vi "Laser Controller.vi"(8 "error in (no error)":errorcluster, 10 "Notifiers":T1, 11 "All Message Queue Cluster":T2) -> (0 "error out":errorcluster)   [LabVIEW 2017]
uses:
  Lib QMH/AllMessageQueue Cluster.ctl
  Lib QMH/Message Cluster.ctl
  Lib Notifier/Notifier.ctl
  PulsePickerValues.ctl
  Lib QMH/MessageQueues.lvlib
  Lib Log/Logging.lvlib
  Lib Notifier/Notifier.lvlib
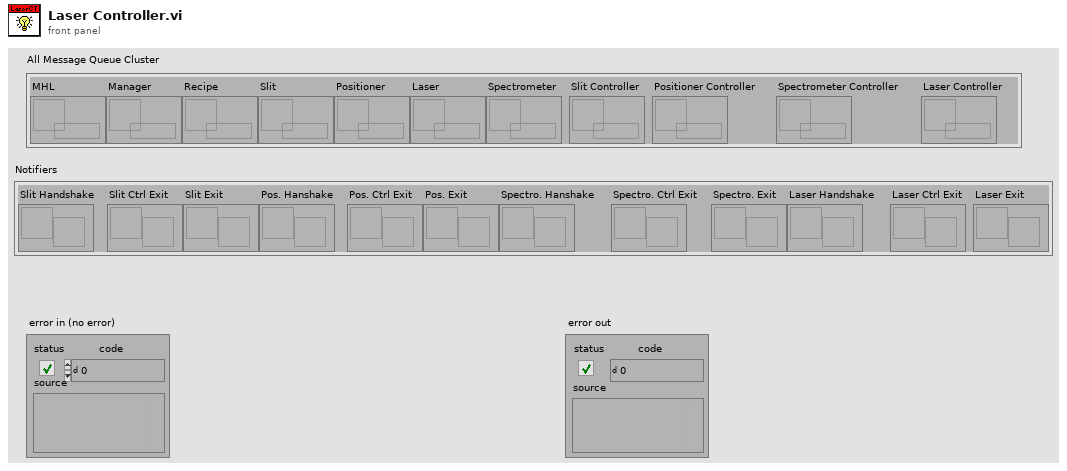
[diagram p1: front panel]
types:
  T1 = typedef "Notifier.lvlib/Notifier.ctl" = cluster{"Slit Handshake":refnum<notifier>, "Slit Ctrl Exit":refnum<notifier>, "Slit Exit":refnum<notifier>, "Pos. Hanshake":refnum<notifier>, "Pos. Ctrl Exit":refnum<notifier>, "Pos. Exit":refnum<notifier>, "Spectro. Hanshake":refnum<notifier>, "Spectro. Ctrl Exit":refnum<notifier>, "Spectro. Exit":refnum<notifier>, "Laser Handshake":refnum<notifier>, "Laser Ctrl Exit":refnum<notifier>, "Laser Exit":refnum<notifier>}
  T2 = typedef "MessageQueues.lvlib/AllMessageQueue Cluster.ctl" = cluster{"MHL":refnum<queue>, "Manager":refnum<queue>, "Recipe":refnum<queue>, "Slit":refnum<queue>, "Positioner":refnum<queue>, "Laser":refnum<queue>, "Spectrometer":refnum<queue>, "Slit Controller":refnum<queue>, "Positioner Controller":refnum<queue>, "Spectrometer Controller":refnum<queue>, "Laser Controller":refnum<queue>}
  T3 = enum16{"open", "replace", "create", "open or create", "replace or create", "replace or create with confirmation"}
  T4 = cluster{"état":bool, "code":i32, "source":string}
  T5 = typedef "PulsePickerValues.ctl" = u16
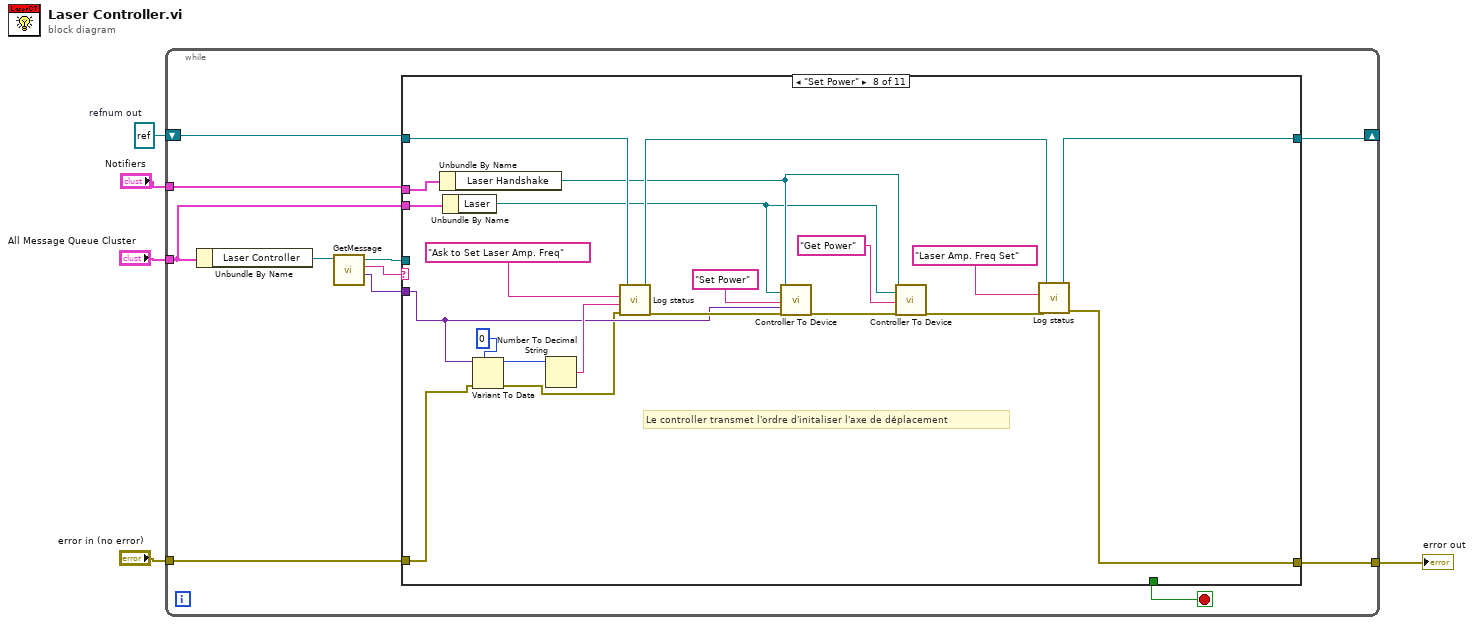
[diagram p0: block diagram]
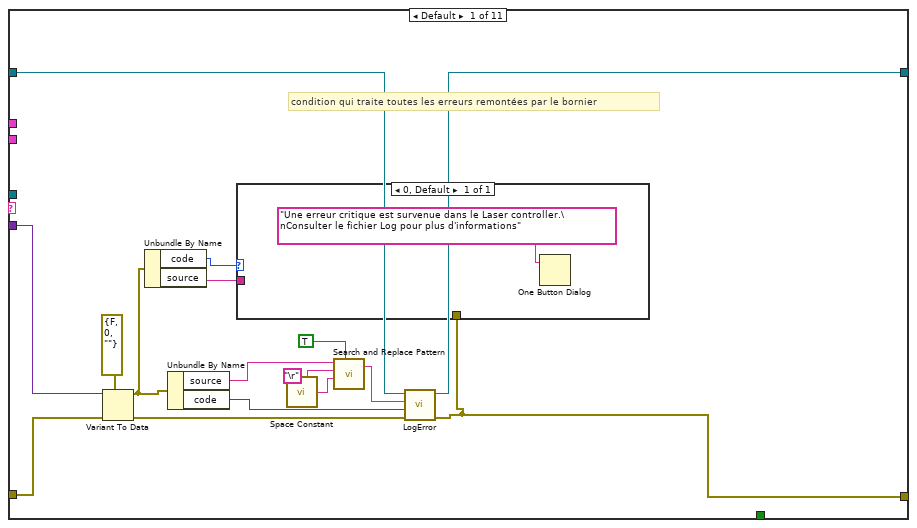
[diagram p2: hidden frame]
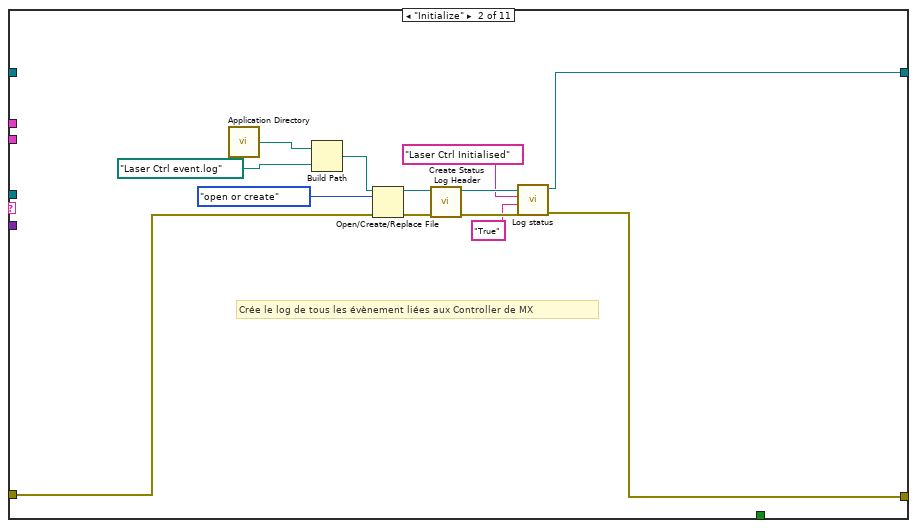
[diagram p3: hidden frame]
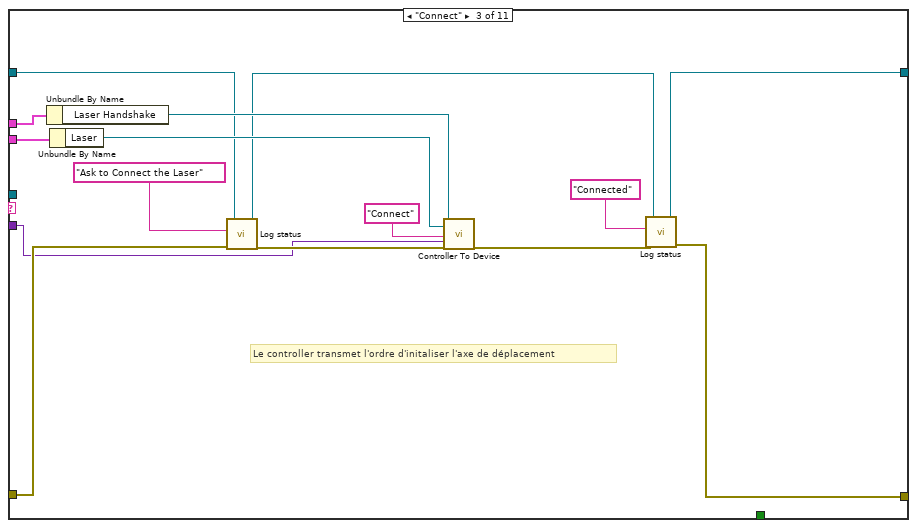
[diagram p4: hidden frame]
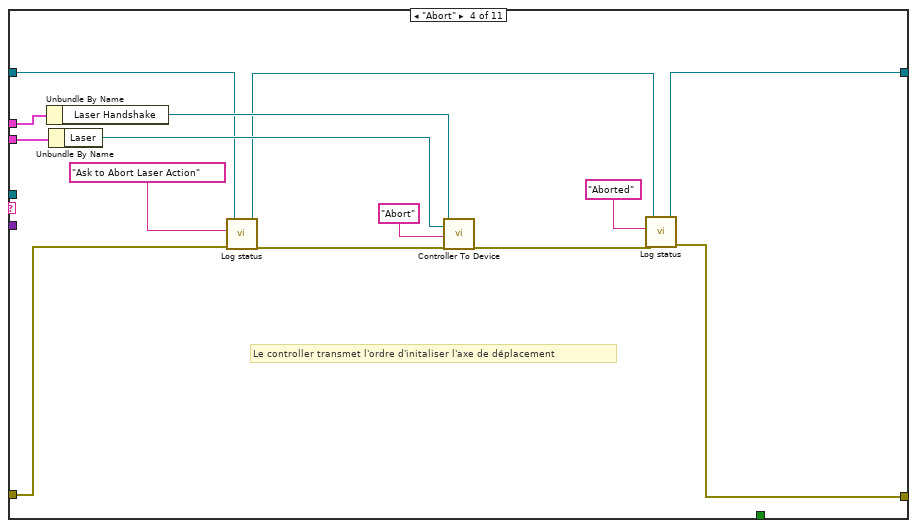
[diagram p5: hidden frame]
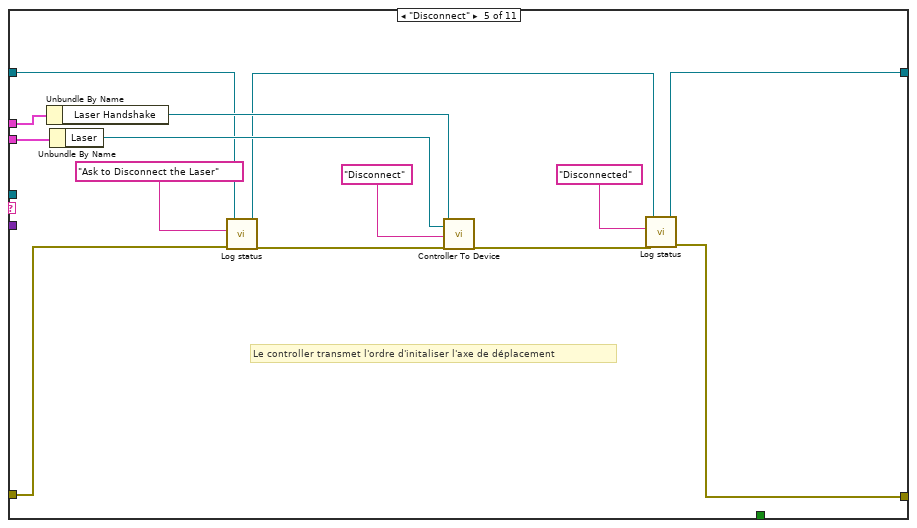
[diagram p6: hidden frame]
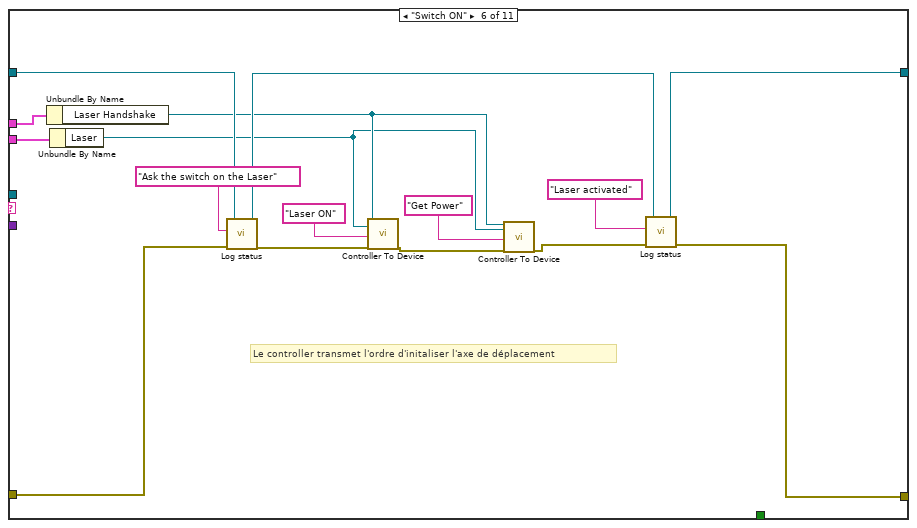
[diagram p7: hidden frame]
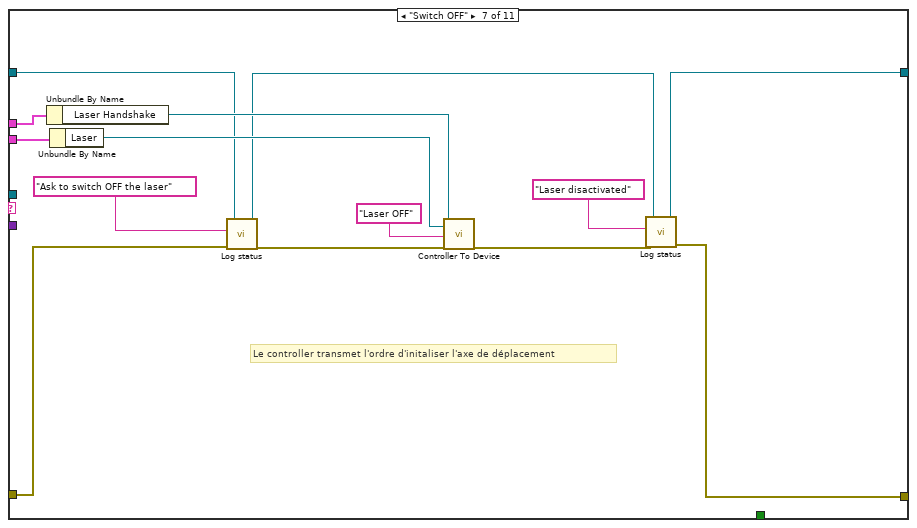
[diagram p8: hidden frame]
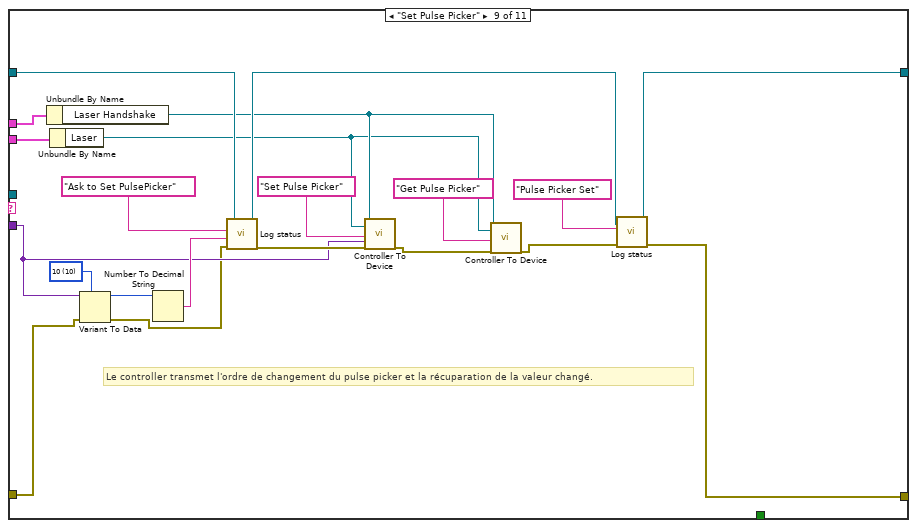
[diagram p9: hidden frame]
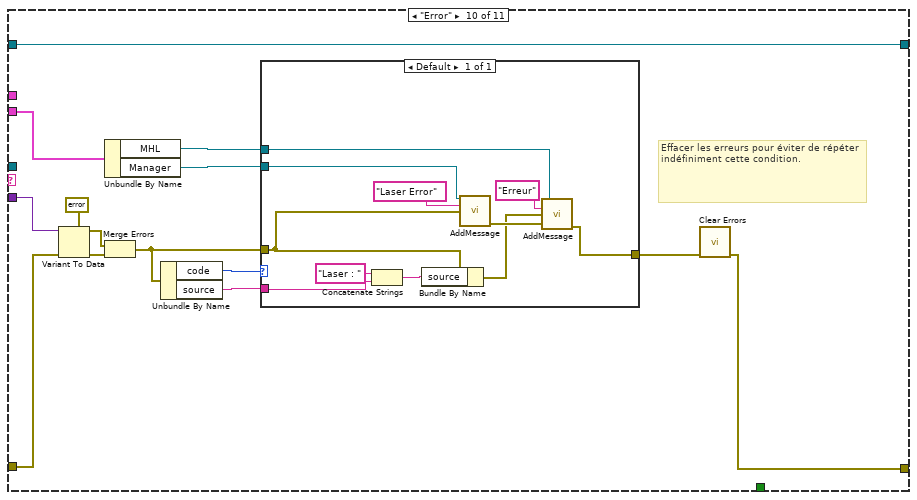
[diagram p10: hidden frame]
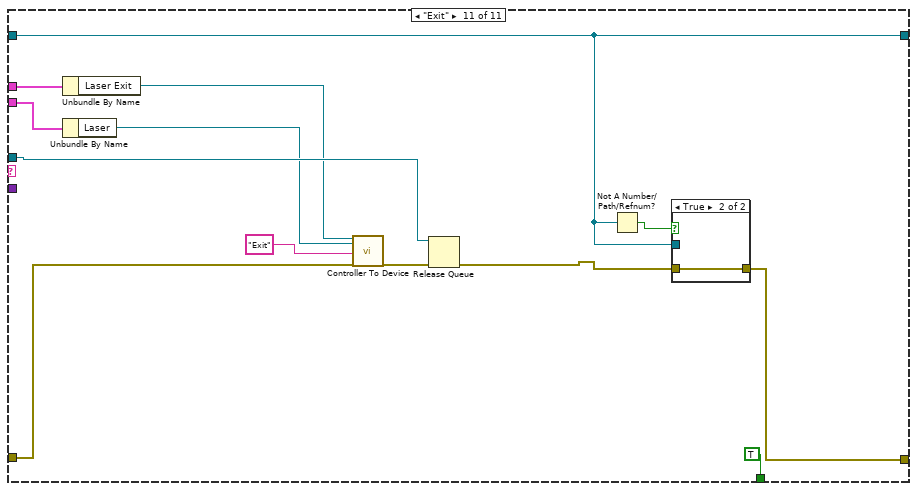
[diagram p11: hidden frame]
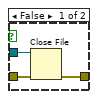
[diagram p12: hidden frame]
diagram:
  w2 = refnum<file> refnum  # refnum out
  n1 = while {
    tunnel: "All Message Queue Cluster" -> [w10]
    tunnel: "Notifiers" -> [w9]
    tunnel: "error in (no error)" -> [w8]
    tunnel: [w15] -> w1
    shift-right: [w12] -> _
    shift-left: w2 -> [w13]
    stop <- w14 stop-if-true
    n2 = Unbundle By Name(w10) -> ("Laser Controller"=w16:refnum<queue>)
    n3 = call "GetMessage.vi"("Message queue"=w16) -> ("Data"=w7:variant, "Message"=w6:string, "Dup Message Queue"=w11:refnum<queue>)  [unwired: 7 in, 1 out]
    n4 = case shown="\"Set Power\"" w6 {
      tunnel: w9 -> [_ _ w61 w75 w89 w105 w119 w140 w161 _ w196]
      tunnel: w10 -> [_ _ w60 w74 w88 w104 w118 w139 w160 w164 w195]
      tunnel: w8 -> [w21 w36 w49 w63 w77 w96 w107 w126 w149 w166 w191]
      tunnel: [_ _ _ _ _ _ _ _ _ _ TRUE] -> w14
      tunnel: w11 -> [_ _ _ _ _ _ _ _ _ _ w197]
      tunnel: w7 -> [w19 _ w47 _ _ _ _ w127 w150 w167 _]
      tunnel: [w17 w34 w52 w66 w80 w99 w110 w134 w155 w175 w193] -> w12
      tunnel: w13 -> [w18 _ w56 w70 w84 w102 w114 w137 w158 w175 w193]
      tunnel: [w20 w35 w54 w68 w82 w101 w112 w136 w157 w165 w194] -> w15
      frame Default {
        # "condition qui traite toutes les erreurs remontées par le bornier"
        n5 = Variant To Data(error in=w21, type=errorcluster {"status"=FALSE, "code"=0, "source"=""} ("error in (no error)"), Variant=w19) -> (data=w32:errorcluster, error out=w23:errorcluster)
        n6 = Unbundle By Name(w32) -> ("code"=w30:i32, "source"=w31:string)
        n7 = Unbundle By Name(w32) -> ("source"=w25:string, "code"=w24:i32)
        n8 = call <vilib>:"Space Constant.vi"() -> ("String"=w27:string)
        n9 = call <vilib>:"Search and Replace Pattern.vi"("string"=w25, "regular expression (\"\")"="\r", "replace string (\"\")"=w27, "replace all? (F)"=TRUE) -> ("result string"=w28:string)  [unwired: 1 in, 1 out]
        n10 = call "LogError.vi"("entrée d'erreur"=w23, "Code"=w24, "Source"=w28, "Error log refnum In"=w18) -> ("error out"=w20:errorcluster, "Error log refnum out"=w17:refnum<file>)  [unwired: 6 in]
        n11 = case shown="0, Default" w30 {
          tunnel: w31 -> [_]
          tunnel: w20 -> [_]
          frame 0, Default {
            n12 = One Button Dialog(message="Une erreur critique est survenue dans le Laser controller.\nConsulter le fichier Log pour plus d'informations" ("chaîne de format")) -> ()  [unwired: 1 in, 1 out]
          }
        }
      }
      frame "Initialize" {
        # "Crée le log de tous les évènement liées aux Controller de MX"
        n13 = call <vilib>:"Application Directory.vi"() -> ("Application Directory"=w43:path)
        n14 = Build Path(base path=w43, name or relative path=path "Laser Ctrl event.log") -> (appended path=w45:path)
        n15 = Open/Create/Replace File(file path (use dialog)=w45, error in=w36, operation (0:open)=T3."open or create" ("opération (0 : open)")) -> (refnum out=w41:refnum<file>, error out=w42:errorcluster)  [unwired: 3 in, 1 out]
        n16 = call "Create Status Log Header.vi"("entrée d'erreur"=w42, "Log File Refnum In"=w41) -> ("sortie d'erreur"=w40:errorcluster, "Log File Refnum out"=w39:refnum<file>)  [unwired: 8 in]
        n17 = call "Log status.vi"("entrée d'erreur"=w40, "Event Data String (-)"="True", "Event string"="Laser Ctrl Initialised", "Log File Refnum In"=w39) -> ("error out"=w35:errorcluster, "Log File Refnum out"=w34:refnum<file>)  [unwired: 6 in]
      }
      frame "Connect" {
        # "Le controller transmet l'ordre d'initaliser l'axe de déplacement"
        n18 = Unbundle By Name(w61) -> ("Laser Handshake"=w59:refnum<notifier>)
        n19 = Unbundle By Name(w60) -> ("Laser"=w58:refnum<queue>)
        n20 = call "Log status.vi"("entrée d'erreur"=w49, "Event string"="Ask to Connect the Laser", "Log File Refnum In"=w56) -> ("error out"=w57:errorcluster, "Log File Refnum out"=w53:refnum<file>)  [unwired: 7 in]
        n21 = call "Controller To Device.vi"("Notifier"=w59, "Message queue"=w58, "Message"="Connect", "Data"=w47, "entrée d'erreur"=w57) -> ("sortie d'erreur"=w55:errorcluster)  [unwired: 12 in, 2 out]
        n22 = call "Log status.vi"("entrée d'erreur"=w55, "Event string"="Connected", "Log File Refnum In"=w53) -> ("error out"=w54:errorcluster, "Log File Refnum out"=w52:refnum<file>)  [unwired: 7 in]
      }
      frame "Abort" {
        # "Le controller transmet l'ordre d'initaliser l'axe de déplacement"
        n23 = Unbundle By Name(w75) -> ("Laser Handshake"=w73:refnum<notifier>)
        n24 = Unbundle By Name(w74) -> ("Laser"=w72:refnum<queue>)
        n25 = call "Log status.vi"("entrée d'erreur"=w63, "Event string"="Ask to Abort Laser Action", "Log File Refnum In"=w70) -> ("error out"=w71:errorcluster, "Log File Refnum out"=w67:refnum<file>)  [unwired: 7 in]
        n26 = call "Controller To Device.vi"("Notifier"=w73, "Message queue"=w72, "Message"="Abort", "entrée d'erreur"=w71) -> ("sortie d'erreur"=w69:errorcluster)  [unwired: 13 in, 2 out]
        n27 = call "Log status.vi"("entrée d'erreur"=w69, "Event string"="Aborted", "Log File Refnum In"=w67) -> ("error out"=w68:errorcluster, "Log File Refnum out"=w66:refnum<file>)  [unwired: 7 in]
      }
      frame "Disconnect" {
        # "Le controller transmet l'ordre d'initaliser l'axe de déplacement"
        n28 = Unbundle By Name(w89) -> ("Laser Handshake"=w87:refnum<notifier>)
        n29 = Unbundle By Name(w88) -> ("Laser"=w86:refnum<queue>)
        n30 = call "Log status.vi"("entrée d'erreur"=w77, "Event string"="Ask to Disconnect the Laser", "Log File Refnum In"=w84) -> ("error out"=w85:errorcluster, "Log File Refnum out"=w81:refnum<file>)  [unwired: 7 in]
        n31 = call "Controller To Device.vi"("Notifier"=w87, "Message queue"=w86, "Message"="Disconnect", "entrée d'erreur"=w85) -> ("sortie d'erreur"=w83:errorcluster)  [unwired: 13 in, 2 out]
        n32 = call "Log status.vi"("entrée d'erreur"=w83, "Event string"="Disconnected", "Log File Refnum In"=w81) -> ("error out"=w82:errorcluster, "Log File Refnum out"=w80:refnum<file>)  [unwired: 7 in]
      }
      frame "Switch ON" {
        # "Le controller transmet l'ordre d'initaliser l'axe de déplacement"
        n33 = Unbundle By Name(w105) -> ("Laser Handshake"=w91:refnum<notifier>)
        n34 = Unbundle By Name(w104) -> ("Laser"=w90:refnum<queue>)
        n35 = call "Log status.vi"("entrée d'erreur"=w96, "Event string"="Ask the switch on the Laser", "Log File Refnum In"=w102) -> ("error out"=w103:errorcluster, "Log File Refnum out"=w100:refnum<file>)  [unwired: 7 in]
        n36 = call "Controller To Device.vi"("Notifier"=w91, "Message queue"=w90, "Message"="Laser ON", "entrée d'erreur"=w103) -> ("sortie d'erreur"=w93:errorcluster)  [unwired: 13 in, 2 out]
        n37 = call "Controller To Device.vi"("Notifier"=w91, "Message queue"=w90, "Message"="Get Power", "entrée d'erreur"=w93) -> ("sortie d'erreur"=w92:errorcluster)  [unwired: 13 in, 2 out]
        n38 = call "Log status.vi"("entrée d'erreur"=w92, "Event string"="Laser activated", "Log File Refnum In"=w100) -> ("error out"=w101:errorcluster, "Log File Refnum out"=w99:refnum<file>)  [unwired: 7 in]
      }
      frame "Switch OFF" {
        # "Le controller transmet l'ordre d'initaliser l'axe de déplacement"
        n39 = Unbundle By Name(w119) -> ("Laser Handshake"=w117:refnum<notifier>)
        n40 = Unbundle By Name(w118) -> ("Laser"=w116:refnum<queue>)
        n41 = call "Log status.vi"("entrée d'erreur"=w107, "Event string"="Ask to switch OFF the laser", "Log File Refnum In"=w114) -> ("error out"=w115:errorcluster, "Log File Refnum out"=w111:refnum<file>)  [unwired: 7 in]
        n42 = call "Controller To Device.vi"("Notifier"=w117, "Message queue"=w116, "Message"="Laser OFF", "entrée d'erreur"=w115) -> ("sortie d'erreur"=w113:errorcluster)  [unwired: 13 in, 2 out]
        n43 = call "Log status.vi"("entrée d'erreur"=w113, "Event string"="Laser disactivated", "Log File Refnum In"=w111) -> ("error out"=w112:errorcluster, "Log File Refnum out"=w110:refnum<file>)  [unwired: 7 in]
      }
      frame "Set Power" {
        # "Le controller transmet l'ordre d'initaliser l'axe de déplacement"
        n44 = Unbundle By Name(w140) -> ("Laser Handshake"=w124:refnum<notifier>)
        n45 = Unbundle By Name(w139) -> ("Laser"=w123:refnum<queue>)
        n46 = Variant To Data(error in=w126, type=u16 0, Variant=w127) -> (data=w129:u16, error out=w125:errorcluster)
        n47 = Number To Decimal String(number=w129) -> (decimal integer string=w128:string)  [unwired: 1 in]
        n48 = call "Log status.vi"("entrée d'erreur"=w125, "Event Data String (-)"=w128, "Event string"="Ask to Set Laser Amp. Freq", "Log File Refnum In"=w137) -> ("error out"=w138:errorcluster, "Log File Refnum out"=w135:refnum<file>)  [unwired: 6 in]
        n49 = call "Controller To Device.vi"("Notifier"=w124, "Message queue"=w123, "Message"="Set Power", "Data"=w127, "entrée d'erreur"=w138) -> ("sortie d'erreur"=w121:errorcluster)  [unwired: 12 in, 2 out]
        n50 = call "Controller To Device.vi"("Notifier"=w124, "Message queue"=w123, "Message"="Get Power", "entrée d'erreur"=w121) -> ("sortie d'erreur"=w120:errorcluster)  [unwired: 13 in, 2 out]
        n51 = call "Log status.vi"("entrée d'erreur"=w120, "Event string"="Laser Amp. Freq Set", "Log File Refnum In"=w135) -> ("error out"=w136:errorcluster, "Log File Refnum out"=w134:refnum<file>)  [unwired: 7 in]
      }
      frame "Set Pulse Picker" {
        w142 = T5 10 items=["80"=80, "40"=40, "20"=20, "10"=10, "0"=0] ("Pulse Picker Set")
        # "Le controller transmet l'ordre de changement du pulse picker et la récuparation de la valeur changé."
        n52 = Unbundle By Name(w161) -> ("Laser Handshake"=w144:refnum<notifier>)
        n53 = Unbundle By Name(w160) -> ("Laser"=w143:refnum<queue>)
        n54 = Variant To Data(error in=w149, type=w142, Variant=w150) -> (data=w141:T5, error out=w148:errorcluster)
        n55 = Number To Decimal String(number=w141) -> (decimal integer string=w151:string)  [unwired: 1 in]
        n56 = call "Log status.vi"("entrée d'erreur"=w148, "Event Data String (-)"=w151, "Event string"="Ask to Set PulsePicker", "Log File Refnum In"=w158) -> ("error out"=w159:errorcluster, "Log File Refnum out"=w156:refnum<file>)  [unwired: 6 in]
        n57 = call "Controller To Device.vi"("Notifier"=w144, "Message queue"=w143, "Message"="Set Pulse Picker", "Data"=w150, "entrée d'erreur"=w159) -> ("sortie d'erreur"=w146:errorcluster)  [unwired: 12 in, 2 out]
        n58 = call "Controller To Device.vi"("Notifier"=w144, "Message queue"=w143, "Message"="Get Pulse Picker", "entrée d'erreur"=w146) -> ("sortie d'erreur"=w145:errorcluster)  [unwired: 13 in, 2 out]
        n59 = call "Log status.vi"("entrée d'erreur"=w145, "Event string"="Pulse Picker Set", "Log File Refnum In"=w156) -> ("error out"=w157:errorcluster, "Log File Refnum out"=w155:refnum<file>)  [unwired: 7 in]
      }
      frame "Error" {
        # "Effacer les erreurs pour éviter de répéter indéfiniment cette condition."
        n60 = Variant To Data(error in=w166, type=T4 {"état"=FALSE, "code"=0, "source"=""} ("sortie d'erreur"), Variant=w167) -> (data=w172:T4, error out=w173:errorcluster)
        n61 = Unbundle By Name(w164) -> ("MHL"=w163:refnum<queue>, "Manager"=w168:refnum<queue>)
        n62 = Merge Errors(w172, w173) -> (w169:errorcluster)
        n63 = Unbundle By Name(w169) -> ("code"=w170:i32, "source"=w162:string)
        n64 = case shown="Default" w170 {
          tunnel: [w184] -> w171
          tunnel: w169 -> [w177]
          tunnel: w168 -> [w181]
          tunnel: w163 -> [w182]
          tunnel: w162 -> [w178]
          frame Default {
            n65 = Concatenate Strings("Laser : " ("string"), w178) -> (w179:string)
            n66 = Bundle By Name(cluster=w177, "source"=w179) -> (w176:errorcluster)
            n67 = call "AddMessage.vi"("Message queue"=w181, "Message"="Laser Error", "Data"=w177) -> ("error out"=w183:errorcluster)  [unwired: 11 in, 1 out]
            n68 = call "AddMessage.vi"("Message queue"=w182, "Message"="Erreur", "Data"=w176, "entrée d'erreur (pas d'erreur)"=w183) -> ("error out"=w184:errorcluster)  [unwired: 10 in, 1 out]
          }
        }
        n69 = call <vilib>:"Clear Errors.vi"("error in (no error)"=w171) -> ("error out"=w165:errorcluster)  [unwired: 5 in, 1 out]
      }
      frame "Exit" {
        n70 = Unbundle By Name(w196) -> ("Laser Exit"=w189:refnum<notifier>)
        n71 = Unbundle By Name(w195) -> ("Laser"=w188:refnum<queue>)
        n72 = call "Controller To Device.vi"("Notifier"=w189, "Message queue"=w188, "Message"="Exit", "entrée d'erreur"=w191) -> ("sortie d'erreur"=w192:errorcluster)  [unwired: 13 in, 2 out]
        n73 = Release Queue(queue=w197, error in (no error)=w192) -> (error out=w187:errorcluster)  [unwired: 1 in, 2 out]
        n74 = Not A Number/Path/Refnum?(number/path/refnum=w193) -> (NaN/Path/Refnum?=w198:bool)
        n75 = case shown="True" w198 {
          tunnel: [w202 w203] -> w194
          tunnel: w187 -> [w201 w203]
          tunnel: w193 -> [w200 _]
          frame False {
            n76 = Close File(refnum=w200, error in=w201) -> (error out=w202:errorcluster)  [unwired: 1 out]
          }
          frame True {
          }
        }
      }
    }
  }
  "error out" <- w1
